vi "zad5.vi"() -> ()   [LabVIEW 2017]
uses:
  <vilib>/express/express analysis/Spectral/Block/exnSpectralBlock spectral measurements RMS poly.vi
  <vilib>/express/express analysis/Spectral/Block/exnSpectralBlock spectral measurements RMS DDT.vi
  <vilib>/express/express analysis/Spectral/XNode/ExpressSpectralMeasurementsBlockNode.xnode
panel:
  in  "Amplituda":dbl(knob) scale=0.0..100.0
  out "Amplituda vs Czêstotliwoœæ":dynamicdata(graph)
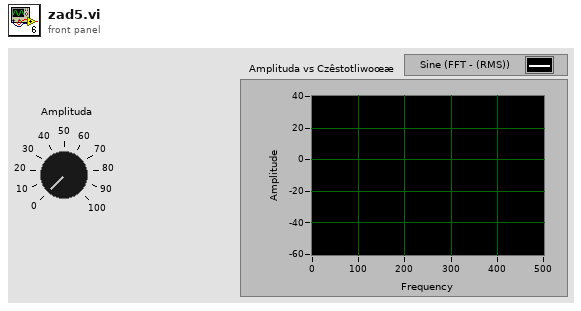
[diagram p1: front panel]
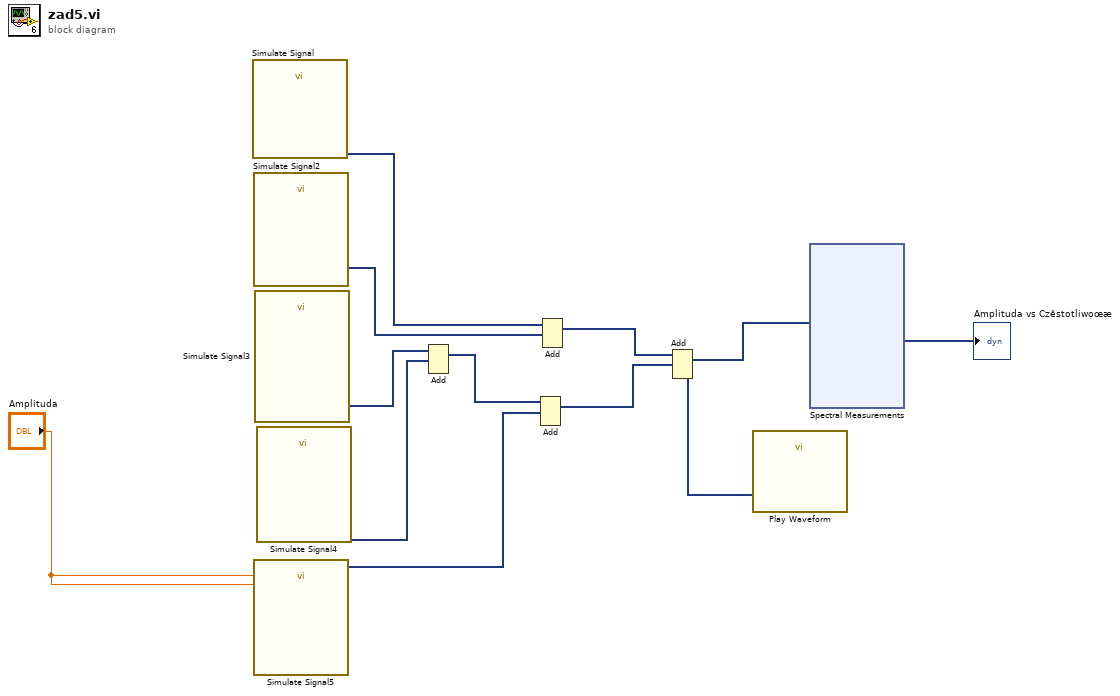
[diagram p0: block diagram]
diagram:
  n1 = call "Simulate Signal"() -> ("Sine"=w11:dynamicdata)  [unwired: 14 in, 1 out]
  n2 = call "Simulate Signal2"() -> ("Sine"=w10:dynamicdata)  [unwired: 14 in, 1 out]
  n3 = call "Simulate Signal5"("Frequency"="Amplituda", "Amplitude"="Amplituda") -> ("Sine with Gamma Noise"=w7:dynamicdata)  [unwired: 12 in, 1 out]
  n4 = call "Simulate Signal3"() -> ("Sawtooth with Poisson Noise"=w9:dynamicdata)  [unwired: 14 in, 1 out]
  n5 = call "Simulate Signal4"() -> ("Sine with MLS Sequence"=w8:dynamicdata)  [unwired: 14 in, 1 out]
  n6 = Add(1:w8, 2:w9) -> (0:w6:dynamicdata)  [unwired: 1 in, 1 out]
  n7 = Add(1:w7, 2:w6) -> (0:w4:dynamicdata)  [unwired: 1 in, 1 out]
  n8 = Add(1:w10, 2:w11) -> (0:w5:dynamicdata)  [unwired: 1 in, 1 out]
  n9 = Add(1:w4, 2:w5) -> (0:w3:dynamicdata)  [unwired: 1 in, 1 out]
  n10 = call "Play Waveform"("Data"=w3) -> ()  [unwired: 18 in, 1 out]
  n11 = xnode "Spectral Measurements"("Signals"=w3) -> ("FFT - (RMS)"=→"Amplituda vs Czêstotliwoœæ":dynamicdata)  [unwired: 1 in, 2 out]
